vi "CoordinateTransform.vi"(0 "input coordiantes":cluster{"x":dbl, "y":dbl}={"x"=0.0, "y"=100.0}, 1 "Conversion Matrix":dbl[][](array[numeric])=[[0.06000000000000002, -8.060365526071922e-18, 3.0], [2.0782800393831513e-17, 0.03999999999999998, 3.9999999999999996]]) -> (2 "output coordiantes":cluster{"x":dbl, "y":dbl}={"x"=2.999999999999999, "y"=7.999999999999998})   [LabVIEW 2011]
uses:
  <vilib>/Analysis/baseanly.llb/A x Vector.vi
  <vilib>/Analysis/NI_AALBase.lvlib
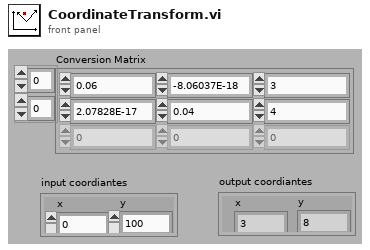
[diagram p1: front panel]
types:
  T1 = cluster{"A x Vector[0]":dbl, "A x Vector[1]":dbl}
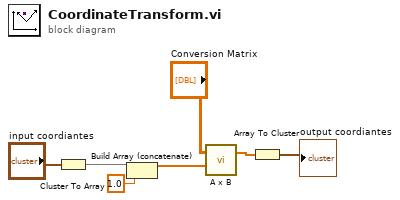
[diagram p0: block diagram]
diagram:
  n1 = Cluster To Array(cluster="input coordiantes") -> (array=w6:dbl[])
  n2 = Build Array (concatenate)(w6, 1.0) -> (w4:dbl[])
  n3 = call-poly <vilib>:"A x B.vi"("Vector"=w4, "A"="Conversion Matrix") -> ("A x Vector"=w2:dbl[])  [unwired: 1 out]
  n4 = Array To Cluster(array=w2) -> (cluster=→"output coordiantes":T1)
